vi "题目5.vi"() -> ()   [LabVIEW 2017]
panel:
  out "显示面板":T1 {"油量" scale=0.0..200.0; "速度（km/h）" scale=0.0..300.0; "转速（r/s）" scale=0.0..8000.0}
  out "油量指示灯":bool=TRUE
  in  "停止":bool
  in  "控制面板":T2 {"档位" scale=0.0..6.0; "油门" scale=0.0..10.0}
  out "时间":dbl
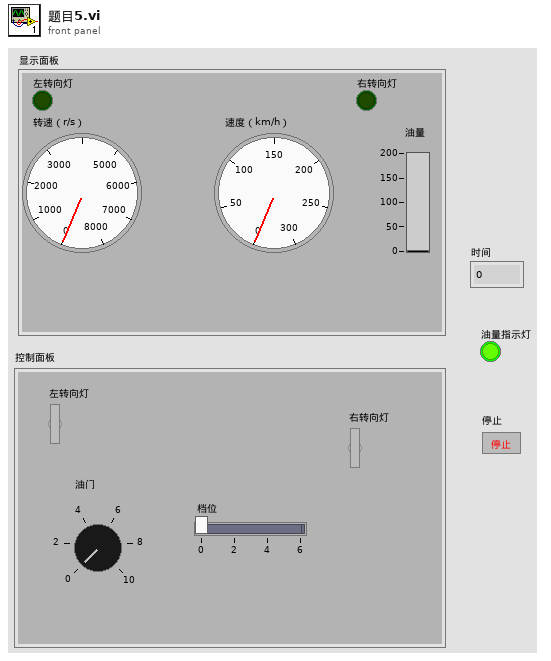
[diagram p1: front panel]
types:
  T1 = cluster{"左转向灯":bool, "右转向灯":bool, "转速（r/s）":dbl, "速度（km/h）":dbl, "油量":dbl}
  T2 = cluster{"油门":dbl, "档位":dbl, "左转向灯":bool, "右转向灯":bool}
  T3 = cluster{"左转向灯":bool, "右转向灯":bool, dbl, dbl, "y":dbl}
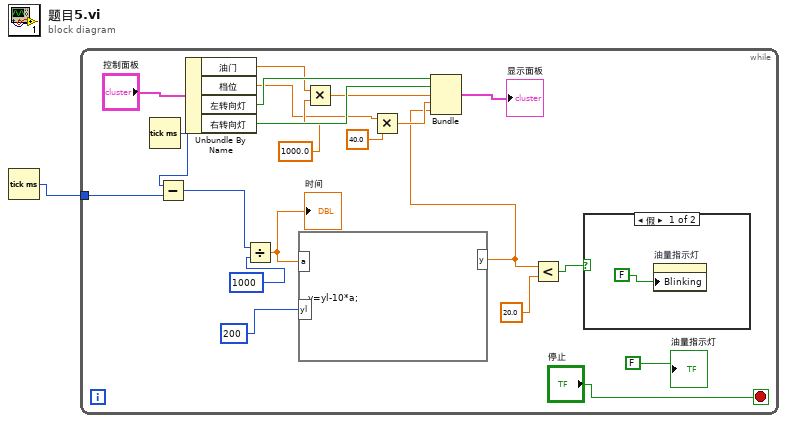
[diagram p0: block diagram]
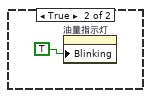
[diagram p2: hidden frame]
diagram:
  n1 = Tick Count (ms)() -> (millisecond timer value=w1:u32)
  n2 = while {
    tunnel: w1 -> [w22]
    stop <- "停止" stop-if-true
    n3 = Tick Count (ms)() -> (millisecond timer value=w21:u32)
    n4 = Subtract(x=w21, y=w22) -> (x-y=w9:u32)
    n5 = Unbundle By Name("控制面板") -> ("油门"=w17:dbl, "档位"=w13:dbl, "左转向灯"=w19:bool, "右转向灯"=w18:bool)
    n6 = Divide(x=w9, y=1000) -> (x/y=w11:dbl)
    "时间" <- w11
    n7 = formula code="y=yl-10*a;"("a"=w11, "yl"=200) -> ("y"=w7:dbl)
    n8 = Multiply(x=w17, y=1000.0) -> (x*y=w15:dbl)
    n9 = Multiply(x=w13, y=40.0) -> (x*y=w12:dbl)
    n10 = Bundle("左转向灯"=w19, "右转向灯"=w18, w15, w12, "y"=w7) -> (→"显示面板":T3)  [unwired: 1 in]
    n11 = Less?(x=w7, y=20.0) -> (x < y?=w2:bool)
    n12 = case shown="假" w2 {
      frame False {
        n13 = property on="油量指示灯" class="Bool (严格)"("Blinking"=FALSE) -> ()  [unwired: 2 in, 2 out]
      }
      frame True {
        n14 = property on="油量指示灯" class="Bool (严格)"("Blinking"=TRUE) -> ()  [unwired: 2 in, 2 out]
      }
    }
    "油量指示灯" <- FALSE
  }
